vi "FdxReadBSPVersionSpecialCvi.vi"(8 "error in":errorcluster, 11 "InstrumentHandle_board in":u32) -> (0 "error out":errorcluster, 1 "BSP Special Version Out":T1, 3 "InstrumentHandle_board out":u32)   [LabVIEW 2020, in "AIM664LV.lvlib"]
doc: "This function returns the version numbers of all board software package components for the AIM board."
uses:
  AIM664LV.lvlib
  AFDX_LibraryAdmin/FdxGlobalDllPath.vi
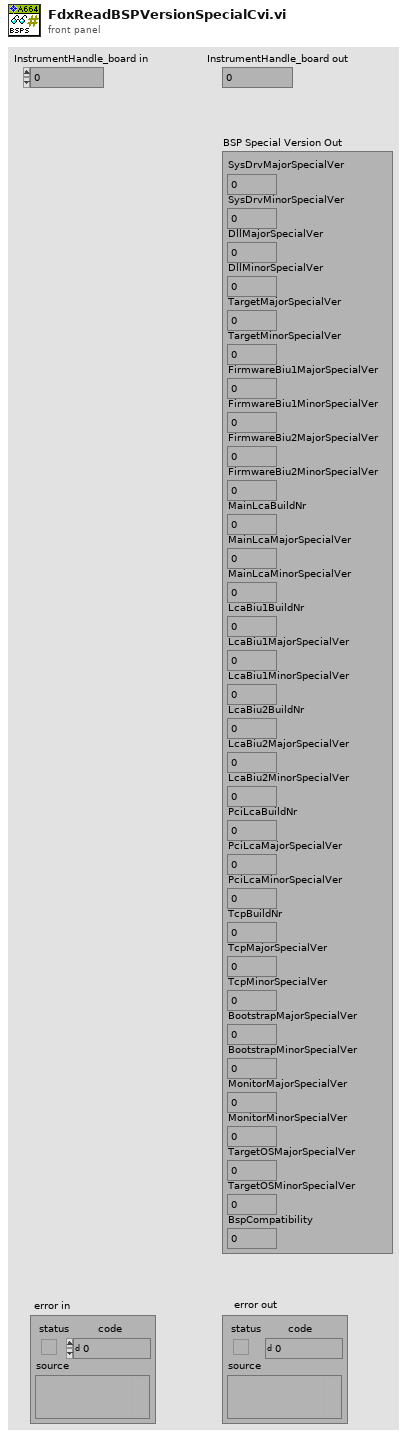
[diagram p1: front panel]
types:
  T1 = cluster{"SysDrvMajorSpecialVer":u32, "SysDrvMinorSpecialVer":u32, "DllMajorSpecialVer":u32, "DllMinorSpecialVer":u32, "TargetMajorSpecialVer":u32, "TargetMinorSpecialVer":u32, "FirmwareBiu1MajorSpecialVer":u32, "FirmwareBiu1MinorSpecialVer":u32, "FirmwareBiu2MajorSpecialVer":u32, "FirmwareBiu2MinorSpecialVer":u32, "MainLcaBuildNr":u32, "MainLcaMajorSpecialVer":u32, "MainLcaMinorSpecialVer":u32, "LcaBiu1BuildNr":u32, "LcaBiu1MajorSpecialVer":u32, "LcaBiu1MinorSpecialVer":u32, "LcaBiu2BuildNr":u32, "LcaBiu2MajorSpecialVer":u32, "LcaBiu2MinorSpecialVer":u32, "PciLcaBuildNr":u32, "PciLcaMajorSpecialVer":u32, "PciLcaMinorSpecialVer":u32, "TcpBuildNr":u32, "TcpMajorSpecialVer":u32, "TcpMinorSpecialVer":u32, "BootstrapMajorSpecialVer":u32, "BootstrapMinorSpecialVer":u32, "MonitorMajorSpecialVer":u32, "MonitorMinorSpecialVer":u32, "TargetOSMajorSpecialVer":u32, "TargetOSMinorSpecialVer":u32, "BspCompatibility":u32}
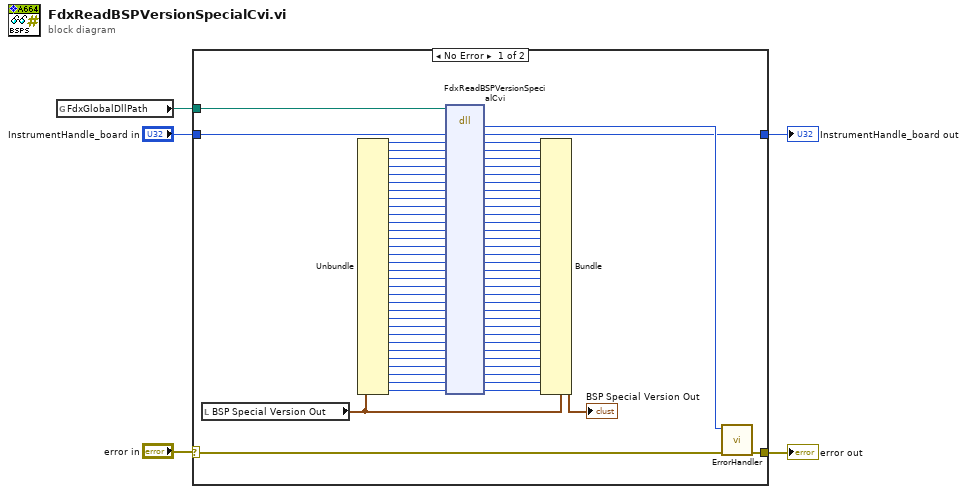
[diagram p0: block diagram]
diagram:
  n1 = global read "FdxGlobalDllPath.vi" "FdxGlobalDllPath"() -> (w3:path)
  n2 = case shown="No Error" "error in" {
    selector: "error in" -> [w76 w79]
    tunnel: [w77 w79] -> w5
    tunnel: w3 -> [w8 _]
    tunnel: "InstrumentHandle_board in" -> [w7 w78]
    tunnel: [w6 w78] -> w1
    frame No Error {
      n3 = local read "BSP Special Version Out"() -> (w9:T1)
      n4 = Unbundle(w9) -> ("SysDrvMajorSpecialVer"=w56:u32, "SysDrvMinorSpecialVer"=w55:u32, "DllMajorSpecialVer"=w54:u32, "DllMinorSpecialVer"=w53:u32, "TargetMajorSpecialVer"=w52:u32, "TargetMinorSpecialVer"=w51:u32, "FirmwareBiu1MajorSpecialVer"=w50:u32, "FirmwareBiu1MinorSpecialVer"=w49:u32, "FirmwareBiu2MajorSpecialVer"=w48:u32, "FirmwareBiu2MinorSpecialVer"=w47:u32, "MainLcaBuildNr"=w46:u32, "MainLcaMajorSpecialVer"=w45:u32, "MainLcaMinorSpecialVer"=w44:u32, "LcaBiu1BuildNr"=w43:u32, "LcaBiu1MajorSpecialVer"=w42:u32, "LcaBiu1MinorSpecialVer"=w41:u32, "LcaBiu2BuildNr"=w40:u32, "LcaBiu2MajorSpecialVer"=w39:u32, "LcaBiu2MinorSpecialVer"=w38:u32, "PciLcaBuildNr"=w37:u32, "PciLcaMajorSpecialVer"=w36:u32, "PciLcaMinorSpecialVer"=w35:u32, "TcpBuildNr"=w34:u32, "TcpMajorSpecialVer"=w33:u32, "TcpMinorSpecialVer"=w32:u32, "BootstrapMajorSpecialVer"=w31:u32, "BootstrapMinorSpecialVer"=w30:u32, "MonitorMajorSpecialVer"=w29:u32, "MonitorMinorSpecialVer"=w28:u32, "TargetOSMajorSpecialVer"=w27:u32, "TargetOSMinorSpecialVer"=w26:u32, "BspCompatibility"=w25:u32)
      n5 = dll-call lib="aim_fdx.19.dll" fn="FdxReadBSPVersionSpecialCvi"(path in=w8, "InstrumentHandle"=w7, "SysDrvMajorSpecialVer"=w56, "SysDrvMinorSpecialVer"=w55, "DllMajorSpecialVer"=w54, "DllMinorSpecialVer"=w53, "TargetMajorSpecialVer"=w52, "TargetMinorSpecialVer"=w51, "FirmwareBiu1MajorSpecialVer"=w50, "FirmwareBiu1MinorSpecialVer"=w49, "FirmwareBiu2MajorSpecialVer"=w48, "FirmwareBiu2MinorSpecialVer"=w47, "MainLcaBuildNr"=w46, "MainLcaMajorSpecialVer"=w45, "MainLcaMinorSpecialVer"=w44, "LcaBiu1BuildNr"=w43, "LcaBiu1MajorSpecialVer"=w42, "LcaBiu1MinorSpecialVer"=w41, "LcaBiu2BuildNr"=w40, "LcaBiu2MajorSpecialVer"=w39, "LcaBiu2MinorSpecialVer"=w38, "PciLcaBuildNr"=w37, "PciLcaMajorSpecialVer"=w36, "PciLcaMinorSpecialVer"=w35, "TcpBuildNr"=w34, "TcpMajorSpecialVer"=w33, "TcpMinorSpecialVer"=w32, "BootstrapMajorSpecialVer"=w31, "BootstrapMinorSpecialVer"=w30, "MonitorMajorSpecialVer"=w29, "MonitorMinorSpecialVer"=w28, "TargetOSMajorSpecialVer"=w27, "TargetOSMinorSpecialVer"=w26, "BspCompatibility"=w25) -> ("status"=w75:i32, "InstrumentHandle"=w6:u32, "SysDrvMajorSpecialVer"=w73:u32, "SysDrvMinorSpecialVer"=w72:u32, "DllMajorSpecialVer"=w71:u32, "DllMinorSpecialVer"=w70:u32, "TargetMajorSpecialVer"=w69:u32, "TargetMinorSpecialVer"=w68:u32, "FirmwareBiu1MajorSpecialVer"=w67:u32, "FirmwareBiu1MinorSpecialVer"=w66:u32, "FirmwareBiu2MajorSpecialVer"=w65:u32, "FirmwareBiu2MinorSpecialVer"=w64:u32, "MainLcaBuildNr"=w63:u32, "MainLcaMajorSpecialVer"=w62:u32, "MainLcaMinorSpecialVer"=w61:u32, "LcaBiu1BuildNr"=w60:u32, "LcaBiu1MajorSpecialVer"=w59:u32, "LcaBiu1MinorSpecialVer"=w58:u32, "LcaBiu2BuildNr"=w57:u32, "LcaBiu2MajorSpecialVer"=w24:u32, "LcaBiu2MinorSpecialVer"=w23:u32, "PciLcaBuildNr"=w22:u32, "PciLcaMajorSpecialVer"=w21:u32, "PciLcaMinorSpecialVer"=w20:u32, "TcpBuildNr"=w19:u32, "TcpMajorSpecialVer"=w18:u32, "TcpMinorSpecialVer"=w17:u32, "BootstrapMajorSpecialVer"=w16:u32, "BootstrapMinorSpecialVer"=w15:u32, "MonitorMajorSpecialVer"=w14:u32, "MonitorMinorSpecialVer"=w13:u32, "TargetOSMajorSpecialVer"=w12:u32, "TargetOSMinorSpecialVer"=w11:u32, "BspCompatibility"=w10:u32)  [unwired: 2 in, 2 out]
      n6 = Bundle(cluster=w9, "SysDrvMajorSpecialVer"=w73, "SysDrvMinorSpecialVer"=w72, "DllMajorSpecialVer"=w71, "DllMinorSpecialVer"=w70, "TargetMajorSpecialVer"=w69, "TargetMinorSpecialVer"=w68, "FirmwareBiu1MajorSpecialVer"=w67, "FirmwareBiu1MinorSpecialVer"=w66, "FirmwareBiu2MajorSpecialVer"=w65, "FirmwareBiu2MinorSpecialVer"=w64, "MainLcaBuildNr"=w63, "MainLcaMajorSpecialVer"=w62, "MainLcaMinorSpecialVer"=w61, "LcaBiu1BuildNr"=w60, "LcaBiu1MajorSpecialVer"=w59, "LcaBiu1MinorSpecialVer"=w58, "LcaBiu2BuildNr"=w57, "LcaBiu2MajorSpecialVer"=w24, "LcaBiu2MinorSpecialVer"=w23, "PciLcaBuildNr"=w22, "PciLcaMajorSpecialVer"=w21, "PciLcaMinorSpecialVer"=w20, "TcpBuildNr"=w19, "TcpMajorSpecialVer"=w18, "TcpMinorSpecialVer"=w17, "BootstrapMajorSpecialVer"=w16, "BootstrapMinorSpecialVer"=w15, "MonitorMajorSpecialVer"=w14, "MonitorMinorSpecialVer"=w13, "TargetOSMajorSpecialVer"=w12, "TargetOSMinorSpecialVer"=w11, "BspCompatibility"=w10) -> (→"BSP Special Version Out":T1)
      n7 = call "ErrorHandler.vi"("error in"=w76, "AIM Error"=w75) -> ("error out"=w77:errorcluster)  [unwired: 9 in]
    }
    frame Error {
    }
  }
  "error out" <- w5
  "InstrumentHandle_board out" <- w1
